vi "make arbitrary waveform_MD.vi"() -> ()   [LabVIEW 2012]
uses:
  Custom Controls/scan mode main settings tab.ctl
  GFG/GFGDisplayRefsGet.vi
  GFG/GFGnumericGet.vi
  GFG/GFGfpRefGet.vi
  GFG/GFGImageRefsGet.vi
  GFG/GFG library.lvlib
  <vilib>/vision/NI_Vision_Development_Module.lvlib
panel:
  out "x = y? 5":bool
  out "x = y? 4":bool
  out "x = y? 3":bool
  out "x = y? 2":bool
  out "x = y?":bool
  out "Source VI":string
  out "error out 3":errorcluster
  out "error out 2":errorcluster
  out "error out":errorcluster
  out "XY Graph 3":cluster{"Y":dbl[], "Y":dbl[]}[](graph)
  out "XY Graph 2":cluster{"Y":dbl[], "Y":dbl[]}[](graph)
  out "XY Graph":cluster{"Y":dbl[], "Y":dbl[]}[](graph)
  out "Waveform Graph 4":dbl[](graph)
  out "Waveform Graph 3":dbl[](graph)
  out "Waveform Graph 2":waveform(dbl)(graph)
  out "Waveform Graph":waveform(dbl)(graph)
  out "size(s) 2":i32
  out "size(s)":i32
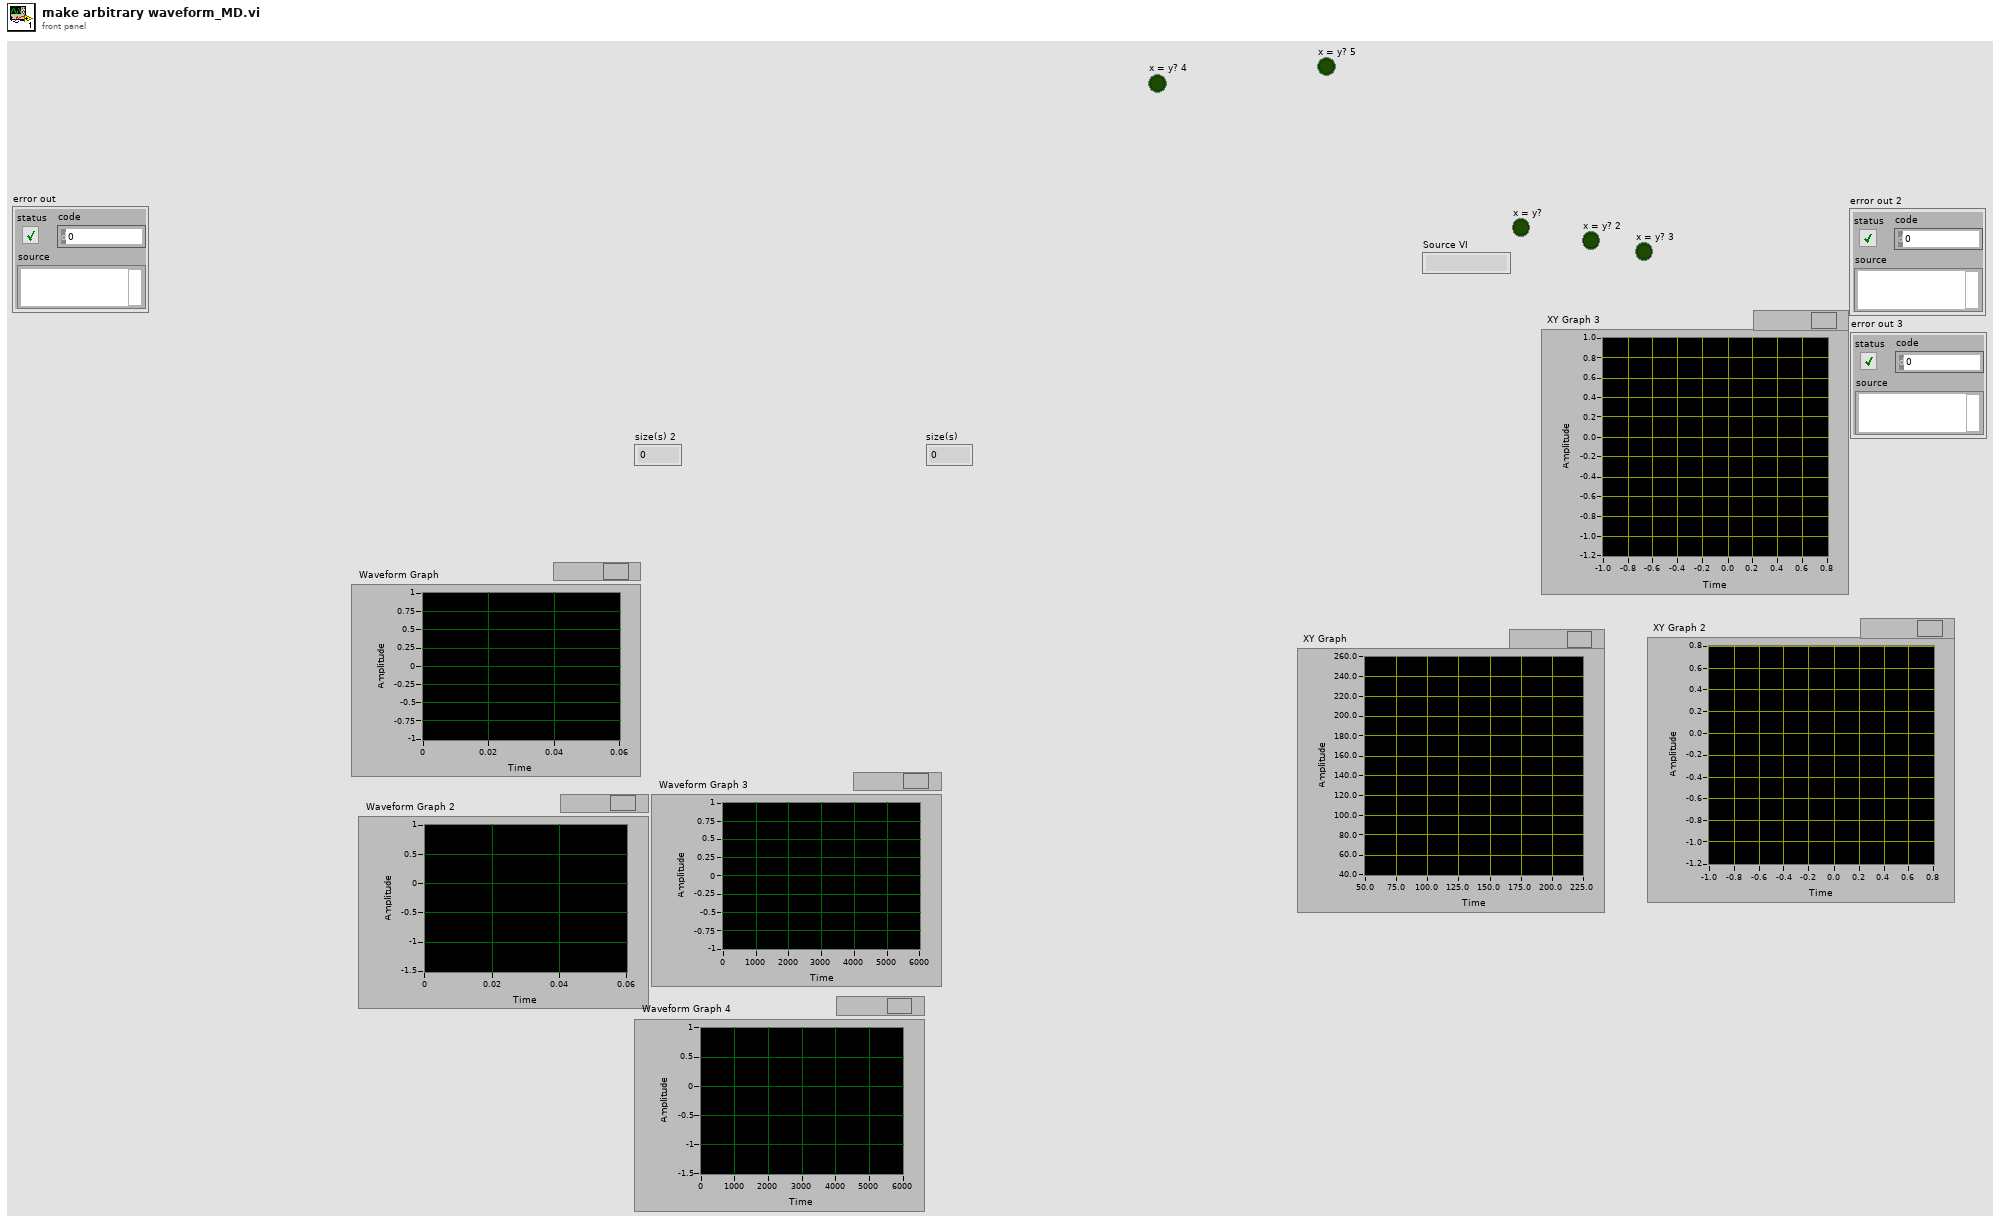
[diagram p1: front panel]
types:
  T1 = cluster{"Channel 1 small":refnum<vi>, "Channel 2 small":refnum<vi>, "Channel 3 small":refnum<vi>, "Channel 4 small":refnum<vi>, "Channel 1 large":refnum<vi>, "Channel 2 large":refnum<vi>, "Channel 3 large":refnum<vi>, "Channel 4 large":refnum<vi>, "RGB overlay":refnum<vi>, "ROI Image display":refnum<vi>, "arb line scan display":refnum<vi>, "Channel 5 large":refnum<vi>}
  T2 = cluster{"xyvoltagefor2frames":dbl[][][], "x.pixels":dbl, "nomin.x.pixels":dbl, "y.pixels":dbl, "fill.fraction":dbl, "x.bidirectional":bool, "y.bidirectional":bool}
  T3 = typedef "ROI Descriptor" = cluster{"Global Rectangle":i32[], "Contours":cluster{"ID":enum32{"External", "Internal"}, "Type":u32, "Coordinates":i32[]}[]}
  T4 = enum8{"Enabled", "Disabled", "Disabled and Grayed Out"}
  T5 = enum32{"Page Enabled", "Page Disabled", "Page Disabled & Grayed"}
  T6 = cluster{"Global Rectangle":i32[], "Contours":cluster{"Contour Type":u32, "ROI Type":u32, "Points":i32[]}[]}
  T7 = typedef "scan mode main settings tab.ctl" = enum32{"2D frame", "2D line scan", "general settings", "Z Stack", "piezo"}
  T8 = cluster{"WaveformChartRef":refnum<vi>, "DigitalRef":refnum<vi>, "ArrayRef":refnum<vi>, "TabControlRef":refnum<vi>, "EnumRef":refnum<vi>, "RingRef":refnum<vi>, "BooleanRef":refnum<vi>, "KnobRef":refnum<vi>, "SlideRef":refnum<vi>, "PathRef":refnum<vi>, "StringRef":refnum<vi>, "ComboBox":refnum<vi>, "WaveformGraphRef":refnum<vi>}
  T9 = typedef "IMAQ Image.ctl" = refnum<image>
  T10 = cluster{"Channel 1 small":T9, "Channel 2 small":T9, "Channel 3 small":T9, "Channel 4 small":T9, "Channel 1 large":T9, "Channel 2 large":T9, "Channel 3 large":T9, "Channel 4 large":T9, "RGB overlay":T9, "ROI Image display":T9, "arb line scan display":T9, "Channel 5 large":T9}
  T11 = cluster{"ID":enum32{"External", "Internal"}, "Type":u32, "Coordinates":i32[]}[]
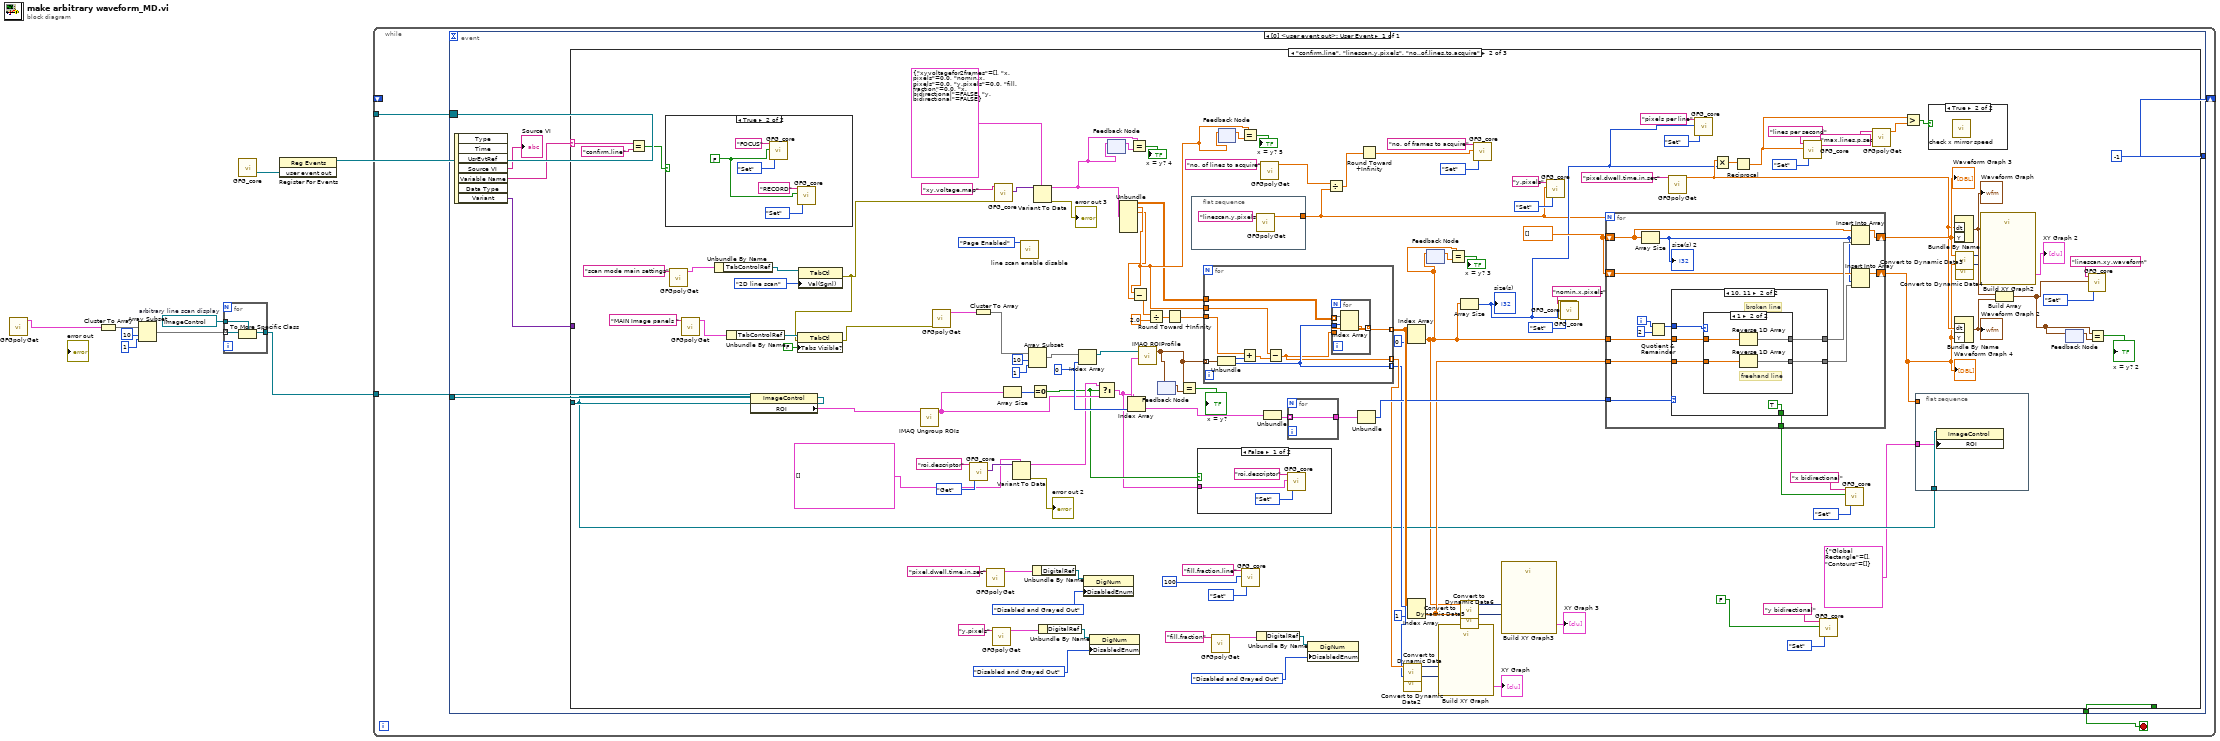
[diagram p0: block diagram]
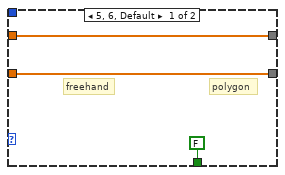
[diagram p6: hidden frame]
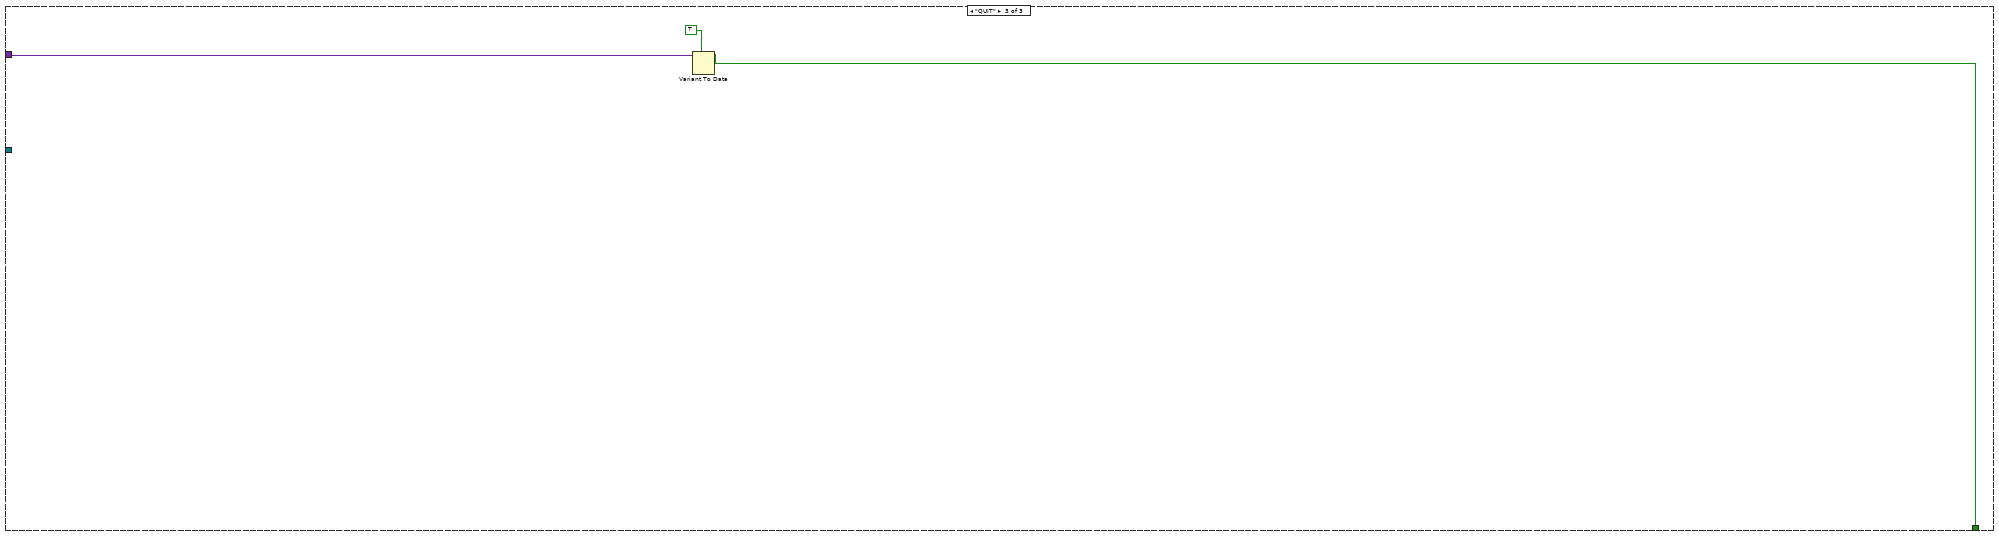
[diagram p8: hidden frame]
diagram:
  w3 = refnum<vi> refnum  # arbitrary line scan display
  n1 = call-poly "GFGpolyGet.vi"() -> ("DisplayRefsOut(generic class)"=w2:T1)  [unwired: 10 in, 1 out]
  n2 = Cluster To Array(cluster=w2) -> (array=w5:refnum<vi>[])
  n3 = Array Subset(array=w5, index=10, length=1) -> (w4:refnum<vi>[])
  n4 = for {
    tunnel: w4 -> [w12] mode=indexing
    tunnel: w3 -> [w11]
    tunnel: [w10] -> w1
    n5 = To More Specific Class(target class=w11, reference=w12) -> (specific class reference=w10:refnum<vi>)  [unwired: 1 in, 1 out]
  }
  n6 = call "GFG_core.vi"() -> ("user event out"=w8:refnum<user-event>)  [unwired: 13 in, 6 out]
  n7 = register-events(w8) -> (reference out=w9:refnum<event-registration>)  [unwired: 2 in, 1 out]
  n8 = while {
    tunnel: w9 -> [w16]
    shift-right: [w14] -> _
    shift-left: _ -> [_]
    tunnel: w1 -> [w13]
    stop <- w15 stop-if-true
    n9 = event shown="[0] <user event out>: User Event" {
      selector: w16 -> [_]
      dyn-events: _ -> [_]
      timeout: _ -> [_]
      tunnel: w13 -> [w22]
      tunnel: [w18] -> w15
      tunnel: [-1 ("length")] -> w14
      event User Event {
        n10 = event-data() -> ("Source VI"=→"Source VI":string, "Variable Name"=w20:string, "Variant"=w19:variant)  [unwired: 1 in, 4 out]
        n11 = case shown="\"confirm.line\", \"linescan.y.pixels\", \"no..of.lines.to.acquire\"" w20 {
          selector: w20 -> [_ w53 _]
          tunnel: w22 -> [_ w92 _]
          tunnel: w19 -> [_ _ w208]
          tunnel: [_ _ w207] -> w18
          frame "False", Default {
          }
          frame "confirm.line", "linescan.y.pixels", "no..of.lines.to.acquire" {
            w49 = 0 ("index")
            w133 = dbl[] []
            n12 = Equal?(x=w53, y="confirm.line") -> (x = y?=w51:bool)
            n13 = case shown="True" w51 {
              frame False {
              }
              frame True {
                w155 = FALSE
                n14 = call "GFG_core.vi"("Variable Name in"="FOCUS", "Variant in"=w155, "Action"=enum16{"Init", "Set", "Get"}."Set") -> ()  [unwired: 10 in, 7 out]
                n15 = call "GFG_core.vi"("Variable Name in"="RECORD", "Variant in"=w155, "Action"=enum16{"Init", "Set", "Get"}."Set") -> ()  [unwired: 10 in, 7 out]
              }
            }
            n16 = call-poly "GFGpolyGet.vi"("Variable Name in"="scan mode main settings") -> ("output cluster"=w106:T8)  [unwired: 9 in, 1 out]
            n17 = call-poly "GFGpolyGet.vi"("Variable Name in"="MAIN Image panels ") -> ("output cluster"=w112:T8)  [unwired: 9 in, 1 out]
            n18 = Unbundle By Name(w106) -> ("TabControlRef"=w108:refnum<vi>)
            n19 = Unbundle By Name(w112) -> ("TabControlRef"=w110:refnum<vi>)
            n20 = property class="ImageControl"(reference=w92) -> ("ROI"=w142:T6)  [unwired: 1 in, 2 out]
            n21 = property class="TabCtl"(reference=w108, "Val(Sgnl)"=scan_mode_main_settings_tab."2D line scan" ("scan mode main settings")) -> (error out=w24:errorcluster)  [unwired: 1 in, 1 out]
            n22 = property class="TabCtl"(reference=w110, error in=w24, "Tabs Visible?"=FALSE) -> (error out=w23:errorcluster)  [unwired: 1 out]
            n23 = call "IMAQ Ungroup ROIs"("ROI Descriptor"=w142) -> ("ROI Descriptors out"=w48:T3[])  [unwired: 3 in, 1 out]
            n24 = call-poly "GFGpolyGet.vi"("error in (no error)"=w23) -> ("Image Refs Out"=w150:T10)  [unwired: 9 in, 1 out]
            n25 = call "GFG_core.vi"("Variable Name in"="roi.descriptor", "Action"=enum16{"Init", "Set", "Get"}."Get") -> ("Variant Out"=w87:variant)  [unwired: 11 in, 6 out]
            n26 = Cluster To Array(cluster=w150) -> (array=w149:T9[])
            n27 = call-poly "GFGpolyGet.vi"("Variable Name in"="pixel.dwell.time.in.sec") -> ("output cluster"=w97:T8)  [unwired: 9 in, 1 out]
            n28 = call-poly "GFGpolyGet.vi"("Variable Name in"="y.pixels") -> ("output cluster"=w55:T8)  [unwired: 9 in, 1 out]
            n29 = call "GFG_core.vi"("Variable Name in"="xy.voltage.map", "error in (no error)"=w24) -> ("Variant Out"=w138:variant)  [unwired: 11 in, 6 out]
            n30 = Array Size(array=w48) -> (size(s)=w88:i32)
            n31 = Variant To Data(type=T3[] [] ("ROI Descriptors out"), Variant=w87) -> (data=w46:T3[], error out=→"error out 2":errorcluster)  [unwired: 1 in]
            n32 = call "line scan enable disable.vi"("Page Enabled State"=T5."Page Enabled") -> ()  [unwired: 11 in]
            n33 = Array Subset(array=w149, index=10, length=1) -> (w145:T9[])
            n34 = Equal To 0?(x=w88) -> (x = 0?=w44:bool)
            n35 = Unbundle By Name(w97) -> ("DigitalRef"=w98:refnum<vi>)
            n36 = Variant To Data(type=T2 {"xyvoltagefor2frames"=[], "x.pixels"=0.0, "nomin.x.pixels"=0.0, "y.pixels"=0.0, "fill.fraction"=0.0, "x.bidirectional"=FALSE, "y.bidirectional"=FALSE} ("output cluster"), Variant=w138) -> (data=w28:T2, error out=→"error out 3":errorcluster)  [unwired: 1 in]
            n37 = Unbundle By Name(w55) -> ("DigitalRef"=w54:refnum<vi>)
            n38 = Index Array(array=w145, index=w49) -> (element=w50:T9)
            n39 = property class="DigNum"(reference=w98, "DisabledEnum"=T4."Disabled and Grayed Out" ("Disabled")) -> ()  [unwired: 1 in, 2 out]
            n40 = property class="DigNum"(reference=w54, "DisabledEnum"=T4."Disabled and Grayed Out" ("Disabled")) -> ()  [unwired: 1 in, 2 out]
            n41 = Select(t=w46, s=w44, f=w48) -> (s? t:f=w43:T3[])
            n42 = feedback #1() -> (w32:T2)  [unwired: 1 in]
            n43 = feedback-in #1(w28) -> ()
            n44 = Unbundle(w28) -> ("xyvoltagefor2frames"=w25:dbl[][][], "x.pixels"=w27:dbl, "nomin.x.pixels"=w26:dbl)  [unwired: 4 out]
            n45 = Index Array(array=w43, index=w49) -> (element=w45:T3)
            n46 = Equal?(x=w28, y=w32) -> (x = y?=→"x = y? 4":bool)
            n47 = Subtract(x=w27, y=w26) -> (x-y=w81:dbl)
            n48 = call "IMAQ ROIProfile"("ROI Descriptor"=w45, "Image"=w50) -> ("Pixel Coordinates"=w42:cluster{"X":u32, "Y":u32}[])  [unwired: 2 in, 4 out]
            n49 = Divide(x=w81, y=2.0) -> (x/y=w79:dbl)
            n50 = feedback-in #2(w42) -> ()
            n51 = feedback #2() -> (w41:cluster{"X":u32, "Y":u32}[])  [unwired: 1 in]
            n52 = Round Toward +Infinity(x=w79) -> (ceil(x): smallest int >= x=w78:dbl)
            n53 = Equal?(x=w42, y=w41) -> (x = y?=→"x = y?":bool)
            n54 = flat-sequence {
              tunnel: [w160] -> w70
              frame #0 {
                n55 = call-poly "GFGpolyGet.vi"("Variable Name in"="linescan.y.pixels") -> ("Numeric"=w160:dbl)  [unwired: 9 in, 1 out]
              }
            }
            n56 = case shown="False" w44 {
              tunnel: w43 -> [w152 _]
              frame False {
                n57 = call "GFG_core.vi"("Variable Name in"="roi.descriptor", "Variant in"=w152, "Action"=enum16{"Init", "Set", "Get"}."Set") -> ()  [unwired: 10 in, 7 out]
              }
              frame True {
              }
            }
            n58 = for {
              tunnel: w42 -> [w201] mode=indexing
              tunnel: [w199] -> w144 mode=indexing
              tunnel: w25 -> [w200]
              tunnel: [w198] -> w140 mode=indexing
              tunnel: [w194] -> w141 mode=indexing
              tunnel: w78 -> [w195]
              tunnel: w27 -> [w193]
              n59 = Unbundle(w201) -> ("X"=w197:u32, "Y"=w198:u32)
              n60 = Add(x=w195, y=w197) -> (x+y=w196:dbl)
              n61 = Subtract(x=w193, y=w196) -> (x-y=w194:dbl)
              n62 = for {
                tunnel: w200 -> [w205] mode=indexing
                tunnel: w194 -> [w204]
                tunnel: w198 -> [w203]
                tunnel: [w202] -> w199 mode=indexing
                n63 = Index Array(array=w205, index (row)=w203, index (col)=w204) -> (element=w202:dbl)
              }
            }
            n64 = call-poly "GFGpolyGet.vi"("Variable Name in"="fill.fraction") -> ("output cluster"=w62:T8)  [unwired: 9 in, 1 out]
            n65 = feedback #3() -> (w31:dbl)  [unwired: 1 in]
            n66 = feedback-in #3(w27) -> ()
            n67 = Equal?(x=w27, y=w31) -> (x = y?=→"x = y? 5":bool)
            n68 = call "GFG_core.vi"("Variable Name in"="fill.fraction.line", "Variant in"=100 ("y"), "Action"=enum16{"Init", "Set", "Get"}."Set") -> ()  [unwired: 10 in, 7 out]
            n69 = Unbundle By Name(w62) -> ("DigitalRef"=w63:refnum<vi>)
            n70 = call-poly "GFGpolyGet.vi"("Variable Name in"="no. of lines to acquire") -> ("Numeric"=w71:dbl)  [unwired: 9 in, 1 out]
            n71 = Unbundle(w45) -> ("Contours"=w147:T11)  [unwired: 1 out]
            n72 = for {
              tunnel: w147 -> [w206] mode=indexing
              tunnel: [w206] -> w146
            }
            n73 = property class="DigNum"(reference=w63, "DisabledEnum"=T4."Disabled and Grayed Out" ("Disabled")) -> ()  [unwired: 1 in, 2 out]
            n74 = Divide(x=w71, y=w70) -> (x/y=w69:dbl)
            n75 = Unbundle(w146) -> ("Type"=w143:u32)  [unwired: 2 out]
            n76 = Round Toward +Infinity(x=w69) -> (ceil(x): smallest int >= x=w68:dbl)
            n77 = call "Convert to Dynamic Data"("Array"=w141) -> ("Dynamic Data Type"=w131:dynamicdata)  [unwired: 3 in]
            n78 = call "Convert to Dynamic Data2"("Array"=w140) -> ("Dynamic Data Type"=w130:dynamicdata)  [unwired: 3 in]
            n79 = Index Array(array=w144, index (col)=0 ("disabled index (col)")) -> (element=w34:dbl[])  [unwired: 1 in]
            n80 = Index Array(array=w144, index (col)=1 ("disabled index (col)")) -> (element=w126:dbl[])  [unwired: 1 in]
            n81 = feedback #4() -> (w36:dbl[])  [unwired: 1 in]
            n82 = feedback-in #4(w34) -> ()
            n83 = call "Build XY Graph"("Y Input"=w130, "X Input"=w131) -> ("XY Graph"=→"XY Graph":cluster{"Y":dbl[], "Y":dbl[]}[])  [unwired: 3 in, 6 out]
            n84 = Equal?(x=w34, y=w36) -> (x = y?=→"x = y? 3":bool)
            n85 = Array Size(array=w34) -> (size(s)=w75:i32)
            "size(s)" <- w75
            n86 = call "Convert to Dynamic Data5"("Array"=w34) -> ("Dynamic Data Type"=w128:dynamicdata)  [unwired: 3 in]
            n87 = call "Convert to Dynamic Data6"("Array"=w126) -> ("Dynamic Data Type"=w129:dynamicdata)  [unwired: 3 in]
            n88 = call "GFG_core.vi"("Variable Name in"="no. of frames to acquire", "Variant in"=w68, "Action"=enum16{"Init", "Set", "Get"}."Set") -> ()  [unwired: 10 in, 7 out]
            n89 = call "Build XY Graph3"("Y Input"=w129, "X Input"=w128) -> ("XY Graph"=→"XY Graph 3":cluster{"Y":dbl[], "Y":dbl[]}[])  [unwired: 3 in, 6 out]
            n90 = call "GFG_core.vi"("Variable Name in"="y.pixels", "Variant in"=w70, "Action"=enum16{"Init", "Set", "Get"}."Set") -> ()  [unwired: 10 in, 7 out]
            n91 = call "GFG_core.vi"() -> ()  [unwired: 13 in, 7 out]
            n92 = call "GFG_core.vi"("Variable Name in"="nomin.x.pixels", "Variant in"=w75, "Action"=enum16{"Init", "Set", "Get"}."Set") -> ()  [unwired: 10 in, 7 out]
            n93 = for {
              N: w70 -> [_]
              tunnel: w126 -> [w175]
              tunnel: w34 -> [w177]
              tunnel: w143 -> [w176]
              shift-right: [w171] -> w117
              shift-left: w133 -> [w166]
              shift-right: [w169] -> w93
              shift-left: w133 -> [w167]
              tunnel: [w164] -> w83
              i -> [w174]
              n94 = Array Size(array=w166) -> (size(s)=w165:i32)
              "size(s) 2" <- w165
              n95 = Quotient & Remainder(x=w174, y=2) -> (x-y*floor(x/y)=w172:i32)  [unwired: 1 out]
              n96 = case shown="10, 11" w176 {
                tunnel: w175 -> [w179 w185]
                tunnel: w177 -> [w180 w186]
                tunnel: [w180 w184] -> w170
                tunnel: [w179 w183] -> w168
                tunnel: w172 -> [_ w182]
                tunnel: [FALSE TRUE] -> w164
                frame 5, 6, Default {
                  # "freehand"
                  # "polygon"
                }
                frame 10, 11 {
                  # "broken line"
                  n97 = case shown="1" w182 {
                    tunnel: w186 -> [w188 w192]
                    tunnel: w185 -> [w187 w191]
                    tunnel: [w188 w190] -> w184
                    tunnel: [w187 w189] -> w183
                    frame 0, Default {
                    }
                    frame 1 {
                      # "freehand line"
                      n98 = Reverse 1D Array(array=w192) -> (reversed array=w190:dbl[])
                      n99 = Reverse 1D Array(array=w191) -> (reversed array=w189:dbl[])
                    }
                  }
                }
              }
              n100 = Insert Into Array(array=w166, index=w165, new element=w170) -> (w171:dbl[])
              n101 = Insert Into Array(array=w167, index=w165, new element=w168) -> (w169:dbl[])
            }
            "Waveform Graph 3" <- w117
            "Waveform Graph 4" <- w93
            n102 = call-poly "GFGpolyGet.vi"("Variable Name in"="pixel.dwell.time.in.sec" ("Tag in")) -> ("Numeric"=w101:dbl)  [unwired: 9 in, 1 out]
            n103 = call "GFG_core.vi"("Variable Name in"="pixels per line", "Variant in"=w75, "Action"=enum16{"Init", "Set", "Get"}."Set") -> ()  [unwired: 10 in, 7 out]
            n104 = Multiply(x=w101, y=w75) -> (x*y=w100:dbl)
            n105 = Reciprocal(x=w100) -> (1/x=w67:dbl)
            n106 = call "GFG_core.vi"("Variable Name in"="lines per second", "Variant in"=w67, "Action"=enum16{"Init", "Set", "Get"}."Set") -> ()  [unwired: 10 in, 7 out]
            n107 = call "GFG_core.vi"("Variable Name in"="y bidirectional", "Variant in"=FALSE, "Action"=enum16{"Init", "Set", "Get"}."Set") -> ()  [unwired: 10 in, 7 out]
            n108 = call "GFG_core.vi"("Variable Name in"="x bidirectional", "Variant in"=w83, "Action"=enum16{"Init", "Set", "Get"}."Set") -> ()  [unwired: 10 in, 7 out]
            n109 = call-poly "GFGpolyGet.vi"("Variable Name in"="max.lines.p.sec") -> ("Numeric"=w65:dbl)  [unwired: 9 in, 1 out]
            n110 = Greater?(x=w67, y=w65) -> (0:w64:bool)
            n111 = flat-sequence {
              tunnel: w93 -> [_]
              tunnel: w92 -> [w163]
              tunnel: T6 {"Global Rectangle"=[], "Contours"=[]} ("ROI") -> [w162]
              frame #0 {
                n112 = property class="ImageControl"(reference=w163, "ROI"=w162) -> ()  [unwired: 1 in, 2 out]
              }
            }
            n113 = case shown="True" w64 {
              frame False {
              }
              frame True {
                n114 = call "check x mirror speed.vi"() -> ()  [unwired: 11 in, 1 out]
              }
            }
            n115 = Bundle By Name("dt"=w101, "Y"=w117) -> (w119:waveform(dbl))  [unwired: 1 in]
            "Waveform Graph" <- w119
            n116 = Bundle By Name("dt"=w101, "Y"=w93) -> (w120:waveform(dbl))  [unwired: 1 in]
            "Waveform Graph 2" <- w120
            n117 = call "Convert to Dynamic Data3"("Array"=w117) -> ("Dynamic Data Type"=w116:dynamicdata)  [unwired: 3 in]
            n118 = call "Convert to Dynamic Data4"("Array"=w93) -> ("Dynamic Data Type"=w115:dynamicdata)  [unwired: 3 in]
            n119 = call "Build XY Graph2"("Y Input"=w115, "X Input"=w116) -> ("XY Graph"=→"XY Graph 2":cluster{"Y":dbl[], "Y":dbl[]}[])  [unwired: 3 in, 6 out]
            n120 = Build Array(w119, w120) -> (w37:waveform(dbl)[])
            n121 = feedback #5() -> (w38:waveform(dbl)[])  [unwired: 1 in]
            n122 = feedback-in #5(w37) -> ()
            n123 = call "GFG_core.vi"("Variable Name in"="linescan.xy.waveform", "Variant in"=w37, "Action"=enum16{"Init", "Set", "Get"}."Set") -> ()  [unwired: 10 in, 7 out]
            n124 = Equal?(x=w37, y=w38) -> (x = y?=→"x = y? 2":bool)
          }
          frame "QUIT" {
            n125 = Variant To Data(type=TRUE, Variant=w208) -> (data=w207:bool)  [unwired: 1 in, 1 out]
          }
        }
      }
    }
  }
